vi "__SET_SP_e4440A.vi"(7 "SP":T1={"start(GHz)"=3.5, "stop(GHz) "=12.5, "BW(MHz)"=8.0, "VBW(Hz)"=1000.0, "ref(dBm)"=-40.0, "log(dB)"=5.0, "AVEG"=10, "AVEG ON/OFF"=FALSE, "Auto Align ON/OFF"=FALSE, "GPIB"="18", "point"=801}) -> ()   [LabVIEW 2017]
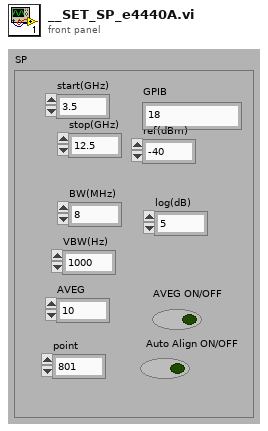
[diagram p1: front panel]
types:
  T1 = cluster{"start(GHz)":dbl, "stop(GHz) ":dbl, "BW(MHz)":dbl, "VBW(Hz)":dbl, "ref(dBm)":dbl, "log(dB)":dbl, "AVEG":i16, "AVEG ON/OFF":bool, "Auto Align ON/OFF":bool, "GPIB":string, "point":i16}
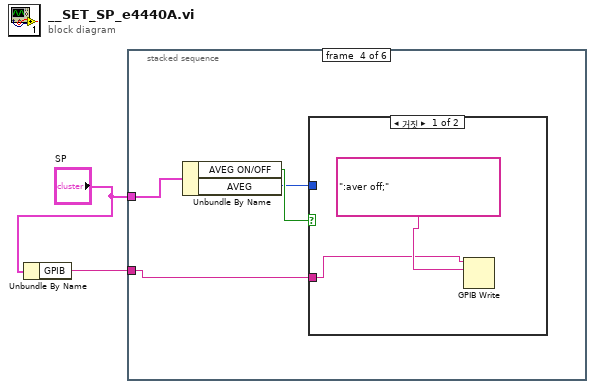
[diagram p0: block diagram]
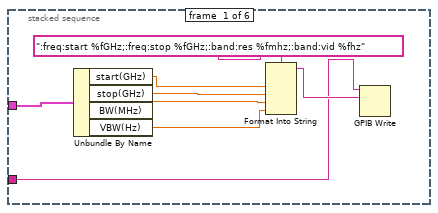
[diagram p2: hidden frame]
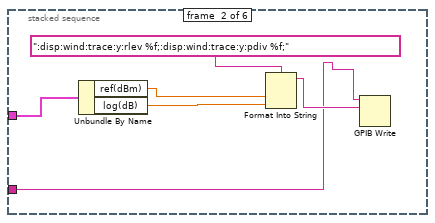
[diagram p3: hidden frame]
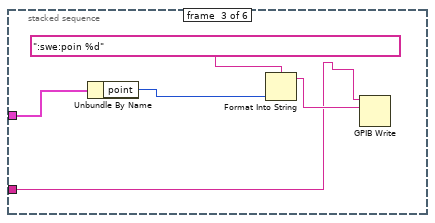
[diagram p4: hidden frame]
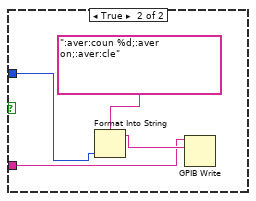
[diagram p5: hidden frame]
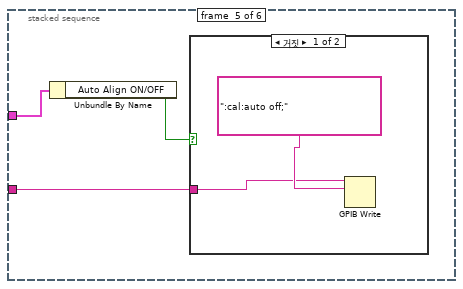
[diagram p6: hidden frame]
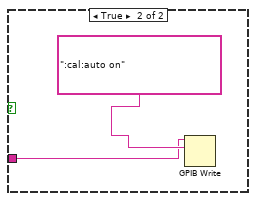
[diagram p7: hidden frame]
diagram:
  n1 = Unbundle By Name("SP") -> ("GPIB"=w1:string)
  n2 = stacked-sequence {
    tunnel: "SP" -> [w9 w15 w20 w25 w34 _]
    tunnel: w1 -> [w4 w11 w17 w22 w32 _]
    frame #0 {
      n3 = Unbundle By Name(w9) -> ("start(GHz)"=w8:dbl, "stop(GHz)"=w6:dbl, "BW(MHz)"=w7:dbl, "VBW(Hz)"=w5:dbl)
      n4 = Format Into String(format string=":freq:start %fGHz;:freq:stop %fGHz;:band:res %fmhz;:band:vid %fhz", w8, w6, w7, w5) -> (resulting string=w10:string)  [unwired: 2 in, 1 out]
      n5 = GPIB Write(0:w4, 1:w10) -> ()  [unwired: 3 in, 2 out]
    }
    frame #1 {
      n6 = Unbundle By Name(w15) -> ("ref(dBm)"=w14:dbl, "log(dB)"=w13:dbl)
      n7 = Format Into String(format string=":disp:wind:trace:y:rlev %f;:disp:wind:trace:y:pdiv %f;", w14, w13) -> (resulting string=w16:string)  [unwired: 2 in, 1 out]
      n8 = GPIB Write(0:w11, 1:w16) -> ()  [unwired: 3 in, 2 out]
    }
    frame #2 {
      n9 = Unbundle By Name(w20) -> ("point"=w19:i16)
      n10 = Format Into String(format string=":swe:poin %d", w19) -> (resulting string=w21:string)  [unwired: 2 in, 1 out]
      n11 = GPIB Write(0:w17, 1:w21) -> ()  [unwired: 3 in, 2 out]
    }
    frame #3 {
      n12 = Unbundle By Name(w25) -> ("AVEG ON/OFF"=w24:bool, "AVEG"=w23:i16)
      n13 = case shown="거짓" w24 {
        tunnel: w23 -> [_ w29]
        tunnel: w22 -> [w26 w28]
        frame False {
          n14 = GPIB Write(0:w26, 1:":aver off;") -> ()  [unwired: 3 in, 2 out]
        }
        frame True {
          n15 = Format Into String(format string=":aver:coun %d;:aver on;:aver:cle", w29) -> (resulting string=w31:string)  [unwired: 2 in, 1 out]
          n16 = GPIB Write(0:w28, 1:w31) -> ()  [unwired: 3 in, 2 out]
        }
      }
    }
    frame #4 {
      n17 = Unbundle By Name(w34) -> ("Auto Align ON/OFF"=w33:bool)
      n18 = case shown="거짓" w33 {
        tunnel: w32 -> [w35 w37]
        frame False {
          n19 = GPIB Write(0:w35, 1:":cal:auto off;") -> ()  [unwired: 3 in, 2 out]
        }
        frame True {
          n20 = GPIB Write(0:w37, 1:":cal:auto on") -> ()  [unwired: 3 in, 2 out]
        }
      }
    }
    frame #5 {
    }
  }
